vi "bmlv_tests__double_dict.vi"() -> ()   [LabVIEW 2014]
uses:
  bmlv/DoubleDictionary/DoubleDictionary.lvclass
panel:
  out "Value":dbl
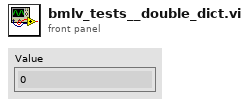
[diagram p1: front panel]
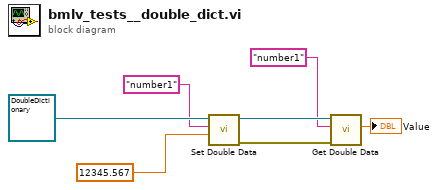
[diagram p0: block diagram]
diagram:
  n1 = call-dynamic "Set Double Data.vi"("Value"=12345.567, "Name"="number1", "DoubleDictionary in"=refnum<class "DoubleDictionary.lvclass"> refnum ("bmlv.lvlib:DoubleDictionary.lvclass")) -> ("error out"=w3:errorcluster, "DoubleDictionary out"=w5:refnum<class "DoubleDictionary.lvclass">)  [unwired: 7 in]
  n2 = call-dynamic "Get Double Data.vi"("error in (no error)"=w3, "Name"="number1", "DoubleDictionary in"=w5) -> ("Value"=→"Value":dbl)  [unwired: 6 in, 2 out]
